vi "GetCurrentXYZPosition (SubVI).vi"(7 ".NET Refnum in - Device":refnum<k24>, 8 "error in (no error)":errorcluster, 11 "Axes Names":string[](array[string])) -> (0 "error out":errorcluster, 1 "Z Position Feedback":dbl, 2 "Y Position Feedback":dbl, 3 "X Position Feedback":dbl, 4 "Current stage position":T1, 5 ".NET Refnum out  - Device":refnum<k24>)   [LabVIEW 2016]
doc: "Returns the Aerotech XYZ stage's current position per axis, or as a cluster with elements X position, Y position, and Z position. The units reflect those of the XYZ stage, so all the lengths are in mm. \n\nBuilt on top of the Aerotech .NET Libraries."
uses:
  C:/Users/Aerotech/Documents/BNL_ThermomechanicalStave/AerotechLibraries/Bin/Aerotech.A3200.dll
  AerotechLibraries/Bin/Aerotech.A3200.dll
panel:
  # "SubVI to retrieve the current position of the XYZ stage"
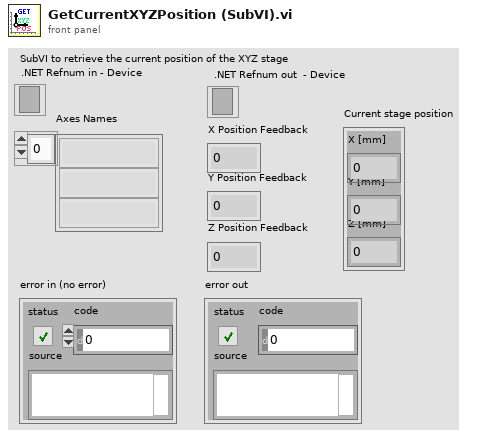
[diagram p1: front panel]
types:
  T1 = cluster{"X [mm]":dbl, "Y [mm]":dbl, "Z [mm]":dbl}
  T2 = typedef "ControllerDiagPacket.ctl" = cluster{"Number of Diag Packets":i32, "Axes":T3[], "error":errorcluster}
  T3 = typedef "AxisDiagPacket.ctl" = cluster{"Axis Name":string, "Analog Input 0":dbl, "Analog Input 1":dbl, "Axis Fault (num)":i32, "Axis Fault (str)":string, "Axis Fault (bits)":cluster{"AmplifierFault":bool, "AmplifierTemperatureFault":bool, "CcwEndOfTravelLimitFault":bool, "CcwSoftwareLimitFault":bool, "CommunicationLostFault":bool, "CwEndOfTravelLimitFault":bool, "CwSoftwareLimitFault":bool, "EmergencyStopFault":bool, "EncoderFault":bool, "ExternalFault":bool, "FeedbackScalingFault":bool, "GantryMisalignFault ":bool, "HallSensorFault":bool, "InPositionTimeoutFault":bool, "MarkerSearchFault":bool, "MaxVelocityCommandFault":bool, "MissedInterruptFault":bool, "MotorTemperatureFault":bool, "None":bool, "OverCurrentFault":bool, "PositionErrorFault":bool, "PositionFeedbackFault":bool, "PowerSupplyFault":bool, "ProbeInputFault":bool, "SafeZoneFault":bool, "VelocityErrorFault":bool, "VelocityFeedbackFault":bool, "VoltageClampFault":bool}, "Axis Status (num)":i32, "Axis Status (str)":string, "Axis Status (bits)":cluster{"BacklashActive":bool, "CalibrationEnabled1D":bool, "CalibrationEnabled2D":bool, "CommandValid":bool, "DriveAbortPending":bool, "DrivePending":bool, "Enabling":bool, "GainMappingEnabled":bool, "GantryAligned":bool, "GantryRealigning":bool, "Homed":bool, "Homing":bool, "IFOVEnabled":bool, "JogGenerating":bool, "Jogging":bool, "JoystickControl":bool, "MasterSlaveControl":bool, "MotionBlocked":bool, "MotionClamped":bool, "MoveDone":bool, "None":bool, "NotVirtual":bool, "Profiling":bool, "Stability0":bool, "Stability1":bool, "TrajectoryFiltering":bool, "WaitDone":bool}, "Current Command":sgl, "Current Error":sgl, "Current Feedback":sgl, "Digital Inputs":i32, "Digital Outputs":i32, "Drive Status":i32, "Drive Status (str)":string, "Drive Status (bits)":cluster{"AccelerationPhase":bool, "AutofocusActive":bool, "BrakeOutput":bool, "CcwEndOfTravelLimitInput":bool, "CosineEncoderError":bool, "CurrentClamp":bool, "CwEndOfTravelLimitInput":bool, "DecelerationPhase":bool, "DualLoopActive":bool, "EmergencyStopInput":bool, "Enabled":bool, "EncoderClipping":bool, "GalvoCalibrationEnabled":bool, "GalvoPowerCorrection":bool, "HallAInput":bool, "HallBInput":bool, "HallCInput":bool, "HighResolutionMode":bool, "HomeLimitInput":bool, "InPosition":bool, "InPosition2":bool, "MarkerInput":bool, "MarkerLatch":bool, "MoveActive":bool, "NoMotorSupply":bool, "None":bool, "PowerLimiting":bool, "ProgrammingFlash":bool, "ProgrammingMXH":bool, "PSOHaltLatch":bool, "ServoControl":bool, "SineEncoderError":bool}, "Position Feedback Auxiliary":dbl, "Position Command":dbl, "Position Error":dbl, "Position Feedback":dbl, "Program Position Command":dbl, "Program Position Error":dbl, "Program Position Feedback":dbl, "Velocity Command":dbl, "Velocity Error":dbl, "Velocity Feedback":dbl}
  T4 = cluster{"Axes Names[0]":string, "Axes Names[1]":string, "Axes Names[2]":string, "Axes Names[3]":string, "Axes Names[4]":string, "Axes Names[5]":string, "Axes Names[6]":string, "Axes Names[7]":string, "Axes Names[8]":string}
  T5 = cluster{"Program Position Feedback":dbl, "Program Position Feedback":dbl, "Program Position Feedback":dbl}
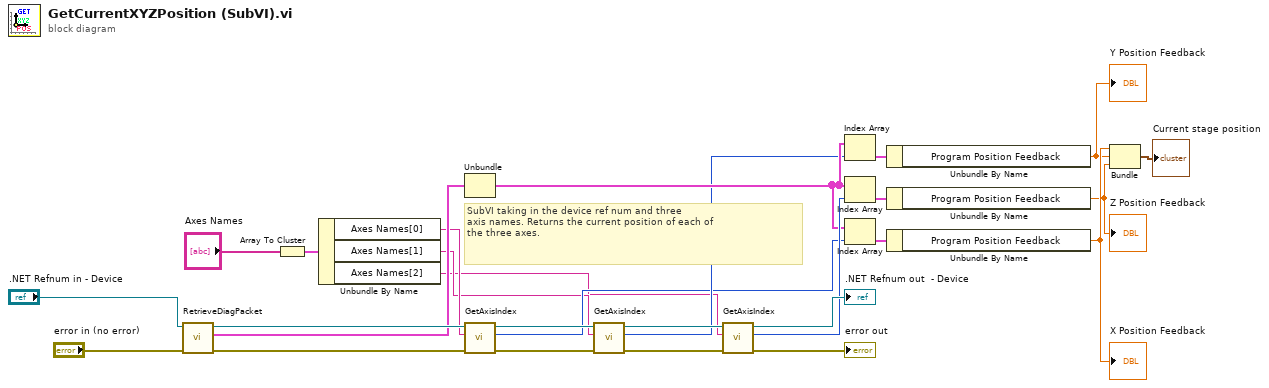
[diagram p0: block diagram]
diagram:
  # "SubVI taking in the device ref num and three\naxis names. Returns the current position of each of\nthe three axes."
  n1 = call "RetrieveDiagPacket.vi"("error in (no error)"="error in (no error)", "Controller In"=".NET Refnum in - Device") -> ("error out"=w11:errorcluster, "ControllerDiagPacket"=w10:T2, "Controller Out"=w17:refnum<k24>)  [unwired: 7 in]
  n2 = Array To Cluster(array="Axes Names") -> (cluster=w8:T4)
  n3 = Unbundle By Name(w8) -> ("Axes Names[0]"=w7:string, "Axes Names[1]"=w6:string, "Axes Names[2]"=w5:string)
  n4 = Unbundle(w10) -> ("Axes"=w22:T3[])  [unwired: 2 out]
  n5 = call "GetAxisIndex.vi"("error in (no error)"=w11, "axis name"=w7, "controller in"=w17) -> ("error out"=w16:errorcluster, "axis index"=w12:i32, "controller out"=w18:refnum<k24>)  [unwired: 6 in]
  n6 = call "GetAxisIndex.vi"("error in (no error)"=w16, "axis name"=w6, "controller in"=w18) -> ("error out"=w23:errorcluster, "axis index"=w15:i32, "controller out"=w26:refnum<k24>)  [unwired: 6 in]
  n7 = call "GetAxisIndex.vi"("error in (no error)"=w23, "axis name"=w5, "controller in"=w26) -> ("error out"=→"error out":errorcluster, "axis index"=w25:i32, "controller out"=→".NET Refnum out  - Device":refnum<k24>)  [unwired: 6 in]
  n8 = Index Array(array=w22, index=w15) -> (element=w14:T3)
  n9 = Index Array(array=w22, index=w25) -> (element=w21:T3)
  n10 = Index Array(array=w22, index=w12) -> (element=w13:T3)
  n11 = Unbundle By Name(w14) -> ("Program Position Feedback"=w3:dbl)
  "Y Position Feedback" <- w3
  n12 = Unbundle By Name(w21) -> ("Program Position Feedback"=w2:dbl)
  "Z Position Feedback" <- w2
  n13 = Unbundle By Name(w13) -> ("Program Position Feedback"=w4:dbl)
  "X Position Feedback" <- w4
  n14 = Bundle("Program Position Feedback"=w4, "Program Position Feedback"=w3, "Program Position Feedback"=w2) -> (→"Current stage position":T5)  [unwired: 1 in]
